vi "Main.vi"() -> ()   [LabVIEW 2020, in "Waveform Generator App.lvclass"]
uses:
  Waveform Generator App.lvclass
  Signal Waveform/Signal Waveform.lvclass
  Signal Waveform/Signal Waveform.lvclass/Signal Waveform.ctl
  Signal Waveform/Write frequency.vi
  Signal Waveform/Write Offset.vi
  Signal Waveform/Write Phase.vi
  Signal Waveform/Write Amplitude.vi
panel:
  out "Waveform Graph 2":waveform(dbl)(graph)
  out "Waveform Graph":waveform(dbl)(graph)
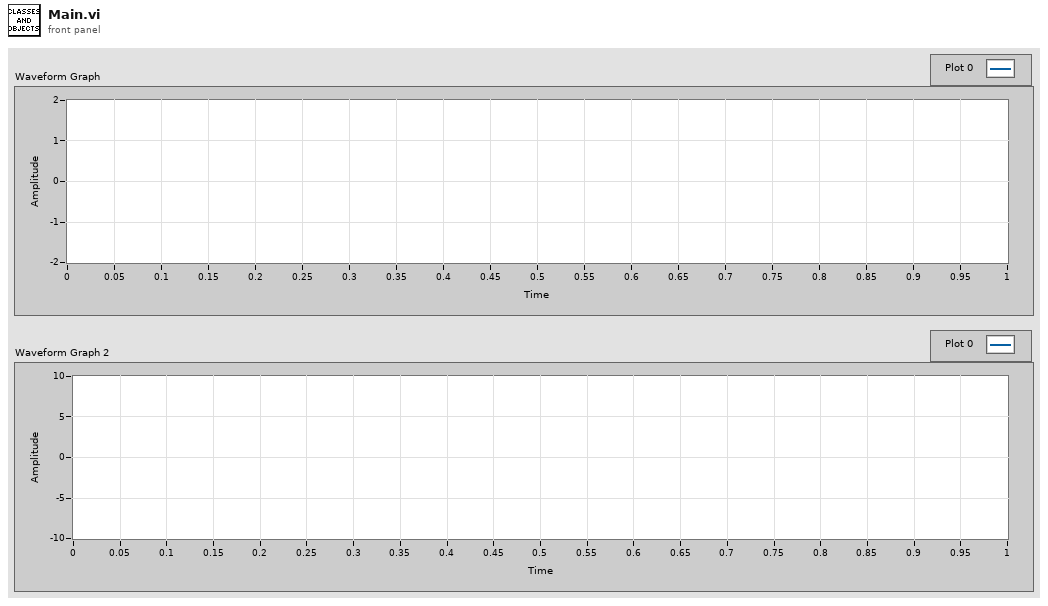
[diagram p1: front panel]
types:
  T1 = enum16{"Sine Wave", "Triangle Wave", "Square Wave", "Sawtooth Wave"}
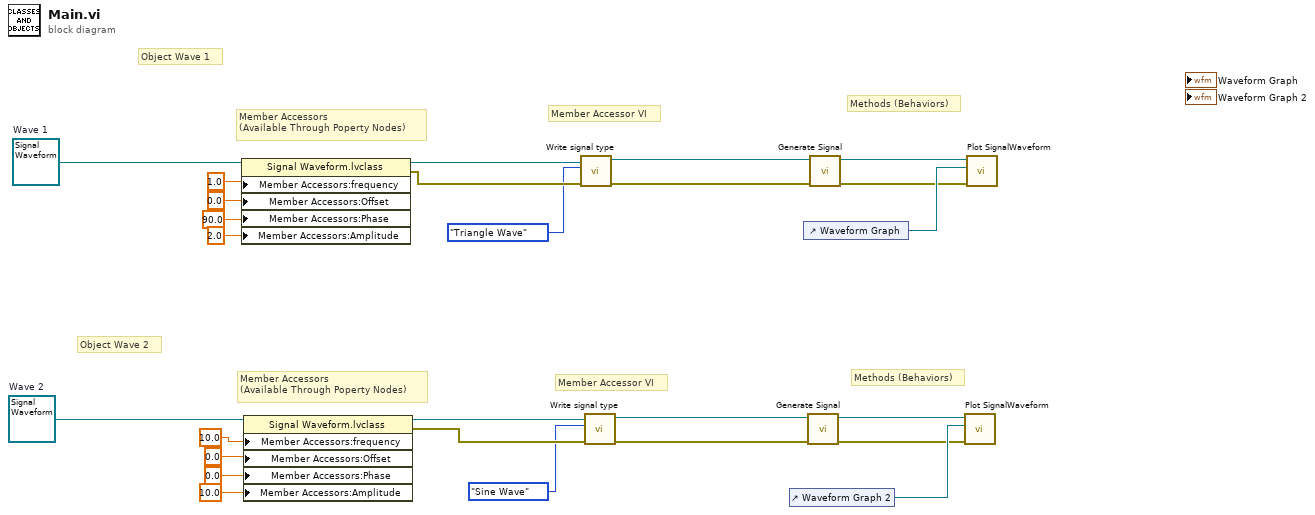
[diagram p0: block diagram]
diagram:
  w25 = refnum<class "Signal Waveform.lvclass"> refnum  # Wave 2
  w26 = refnum<class "Signal Waveform.lvclass"> refnum  # Wave 1
  # "Methods (Behaviors)"
  # "Methods (Behaviors)"
  # "Member Accessor VI"
  # "Member Accessor VI"
  # "Member Accessors\n(Available Through Poperty Nodes)"
  # "Member Accessors\n(Available Through Poperty Nodes)"
  # "Object Wave 2"
  # "Object Wave 1"
  n1 = property class="Signal Waveform.lvclass"(reference=w26, "Member Accessors:frequency"=1.0 ("Offset"), "Member Accessors:Offset"=0.0 ("frequency"), "Member Accessors:Phase"=90.0 ("Phase"), "Member Accessors:Amplitude"=2.0 ("Amplitude")) -> (reference out=w4:refnum<class "Signal Waveform.lvclass">, error out=w10:errorcluster)  [unwired: 1 in]
  n2 = property class="Signal Waveform.lvclass"(reference=w25, "Member Accessors:frequency"=10.0 ("Offset"), "Member Accessors:Offset"=0.0 ("frequency"), "Member Accessors:Phase"=0.0 ("Phase"), "Member Accessors:Amplitude"=10.0 ("Amplitude")) -> (reference out=w7:refnum<class "Signal Waveform.lvclass">, error out=w11:errorcluster)  [unwired: 1 in]
  n3 = call "Write signal type.vi"("error in (no error)"=w10, "signal type"=T1."Triangle Wave", "Signal Waveform in"=w4) -> ("error out"=w5:errorcluster, "Signal Waveform out"=w1:refnum<class "Signal Waveform.lvclass">)  [unwired: 7 in]
  n4 = call "Write signal type.vi"("error in (no error)"=w11, "signal type"=T1."Sine Wave", "Signal Waveform in"=w7) -> ("error out"=w8:errorcluster, "Signal Waveform out"=w6:refnum<class "Signal Waveform.lvclass">)  [unwired: 7 in]
  n5 = control-ref of="Waveform Graph 2"() -> (w13:refnum<vi>)
  n6 = control-ref of="Waveform Graph"() -> (w14:refnum<vi>)
  n7 = call "Generate Signal.vi"("error in (no error)"=w8, "Signal Waveform in"=w6) -> ("error out"=w12:errorcluster, "Signal Waveform out"=w15:refnum<class "Signal Waveform.lvclass">)  [unwired: 8 in]
  n8 = call "Generate Signal.vi"("error in (no error)"=w5, "Signal Waveform in"=w1) -> ("error out"=w9:errorcluster, "Signal Waveform out"=w16:refnum<class "Signal Waveform.lvclass">)  [unwired: 8 in]
  n9 = call "Plot SignalWaveform.vi"("error in (no error)"=w12, "WFGraph Refnum"=w13, "Signal Waveform in"=w15) -> ()  [unwired: 7 in, 2 out]
  n10 = call "Plot SignalWaveform.vi"("error in (no error)"=w9, "WFGraph Refnum"=w14, "Signal Waveform in"=w16) -> ()  [unwired: 7 in, 2 out]
